vi "Render TDMS Metatdata.vi"(8 "error in":errorcluster, 11 "File Path":path) -> (0 "error out":errorcluster, 2 "Wiki entry":string, 3 "Rendered metadata":string)   [LabVIEW 2020]
panel:
  out "first subarray":string[](array[string])
  out "group/channel names":string[][](array[string])
  out "property values":variant[](array[variant])
  out "property names":string[](array[string])
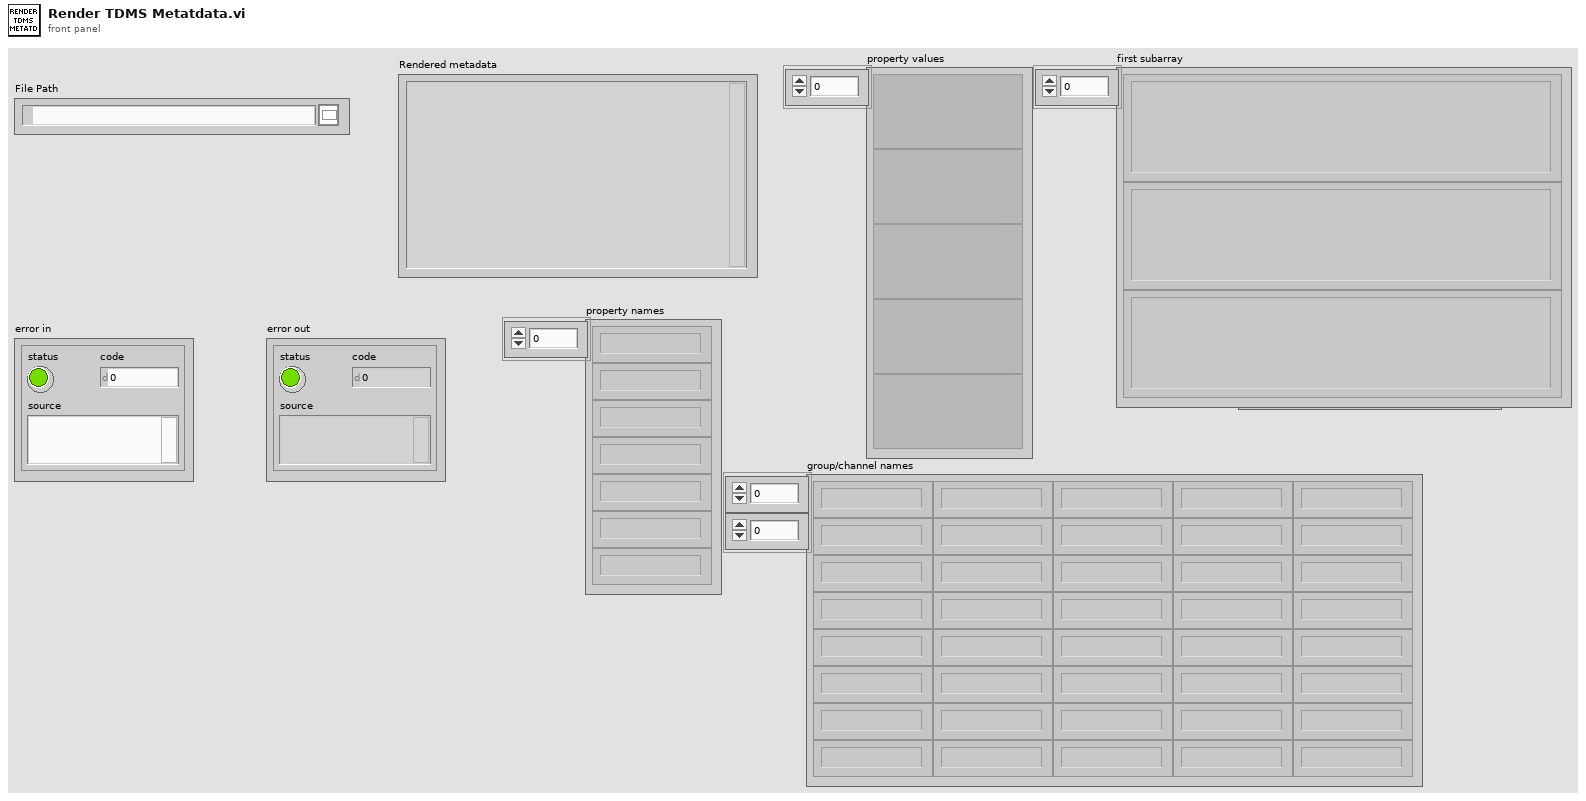
[diagram p1: front panel]
types:
  T1 = enum16{"open", "open or create", "create or replace", "create", "open (read-only)"}
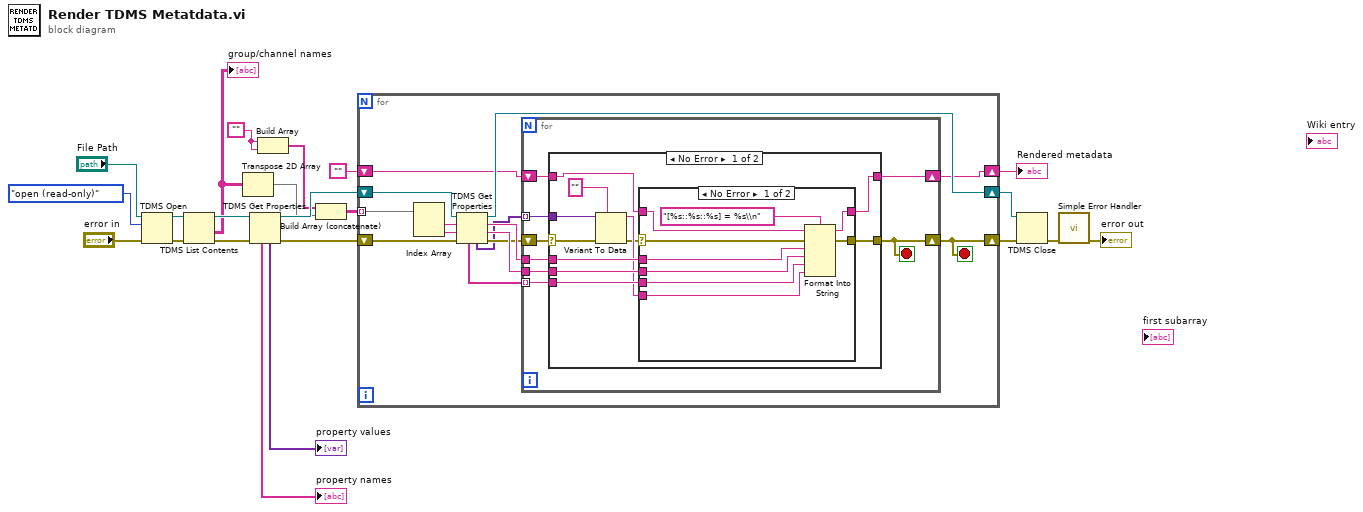
[diagram p0: block diagram]
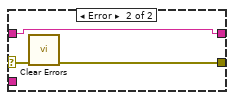
[diagram p2: hidden frame]
diagram:
  w5 = ""
  n1 = TDMS Open(8:"error in", 10:T1."open (read-only)" ("operation (0:open)"), 11:"File Path") -> (0:w16:errorcluster, 3:w14:refnum<k34>)  [unwired: 4 in]
  n2 = TDMS List Contents(4:w16, 7:w14) -> (0:w15:errorcluster, 1:w3:string[][], 3:w13:refnum<k34>)  [unwired: 1 in, 1 out]
  "group/channel names" <- w3
  n3 = Transpose 2D Array(2D array=w3) -> (transposed array=w2:string[][])
  n4 = TDMS Get Properties(8:w15, 11:w13) -> (0:w11:errorcluster, 3:w12:refnum<k34>, 4:→"property values":variant[], 6:→"property names":string[])  [unwired: 4 in, 2 out]
  n5 = Build Array(w5, w5) -> (w4:string[])
  n6 = Build Array (concatenate)(w4, w2) -> (w1:string[][])
  n7 = for {
    tunnel: w1 -> [w36] mode=indexing
    shift-right: [w31] -> w10
    shift-left: w12 -> [w33]
    shift-right: [w23] -> w9
    shift-left: w11 -> [w32]
    shift-right: [w25] -> w7
    shift-left: "" -> [w26]
    stop <- w23 stop-if-true
    n8 = Index Array(array=w36) -> (element #1=w35:string, element #2=w34:string)  [unwired: 2 in]
    n9 = TDMS Get Properties(8:w32, 9:w34, 10:w35, 11:w33) -> (0:w28:errorcluster, 1:w29:string, 2:w30:string, 3:w31:refnum<k34>, 4:w24:variant[], 6:w27:string[])  [unwired: 2 in]
    n10 = for {
      tunnel: w30 -> [w44]
      tunnel: w29 -> [w43]
      tunnel: w27 -> [w42] mode=indexing
      shift-right: [w38] -> w23
      shift-left: w28 -> [w39]
      shift-right: [w37] -> w25
      shift-left: w26 -> [w41]
      tunnel: w24 -> [w40] mode=indexing
      stop <- w38 stop-if-true
      n11 = case shown="No Error" w39 {
        selector: w39 -> [w45 w69]
        tunnel: w44 -> [w55 _]
        tunnel: w43 -> [w54 _]
        tunnel: [w53 w69] -> w38
        tunnel: w42 -> [w52 _]
        tunnel: w41 -> [w51 w68]
        tunnel: [w50 w68] -> w37
        tunnel: w40 -> [w49 _]
        frame No Error {
          n12 = Variant To Data(error in=w45, type="", Variant=w49) -> (data=w47:string, error out=w46:errorcluster)
          n13 = case shown="No Error" w46 {
            selector: w46 -> [w57 w66]
            tunnel: w55 -> [w64 _]
            tunnel: w54 -> [w63 _]
            tunnel: [w62 w65] -> w53
            tunnel: w52 -> [w61 _]
            tunnel: w51 -> [w60 w67]
            tunnel: [w59 w67] -> w50
            tunnel: w47 -> [w58 _]
            frame No Error {
              n14 = Format Into String(format string="[%s::%s::%s] = %s\\n", initial string=w60, error in=w57, w64, w63, w61, w58) -> (resulting string=w59:string, error out=w62:errorcluster)
            }
            frame Error {
              n15 = call <vilib>:"Clear Errors.vi"("error in (no error)"=w66) -> ("error out"=w65:errorcluster)  [unwired: 5 in, 1 out]
            }
          }
        }
        frame Error {
        }
      }
    }
  }
  "Rendered metadata" <- w7
  n16 = TDMS Close(8:w9, 11:w10) -> (0:w19:errorcluster)  [unwired: 1 out]
  n17 = call <vilib>:"Simple Error Handler.vi"("error in (no error)"=w19) -> ("error out"=→"error out":errorcluster)  [unwired: 4 in, 4 out]
